vi "Coord window-PictureMap zoom to fit.vi"(8 "error in":errorcluster, 10 "Conditional?":bool) -> (0 "error out":errorcluster)   [LabVIEW 2013]
uses:
  Globals/Coord window-Globals.vi
panel:
  # "ZOOM TO FIT"
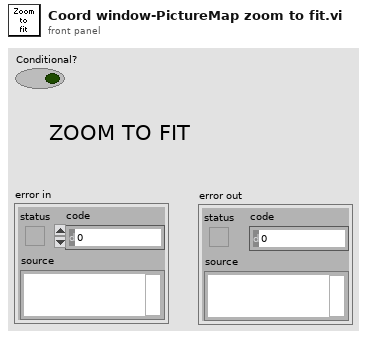
[diagram p1: front panel]
types:
  T1 = typedef "Coordinate list window refs.ctl" = cluster{"Window Name (i.e. Key)":string, "menu reference":refnum<k9>, "VI's reference":refnum<vi>, "Pane 1":refnum<vi>, "Pane 2":refnum<vi>, "Coord Listbox":refnum<vi>, "File name":refnum<vi>, "Picture Map":refnum<vi>, "Stage XYZ Position ind.":refnum<vi>}
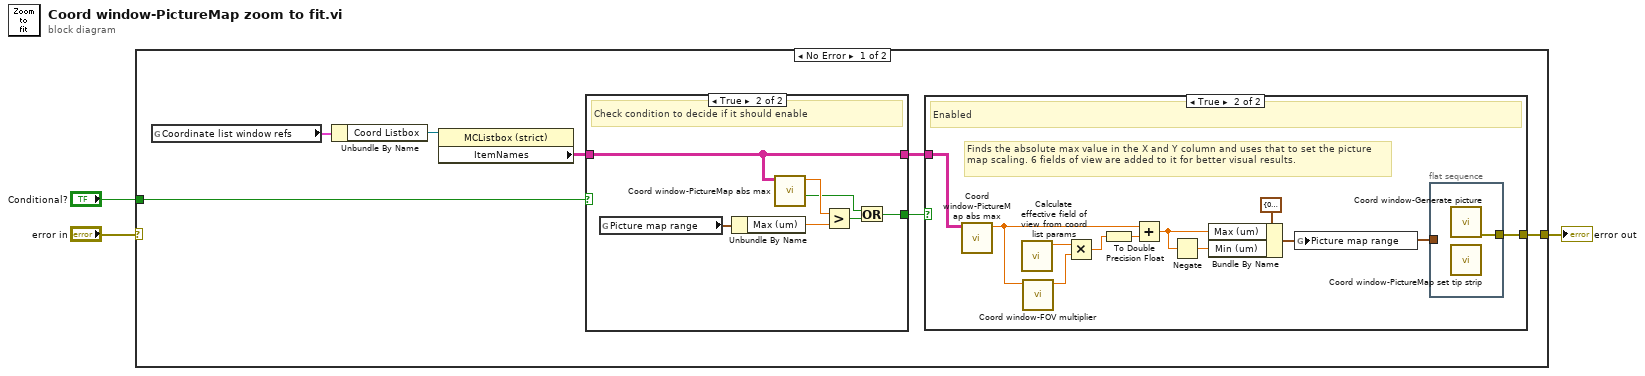
[diagram p0: block diagram]
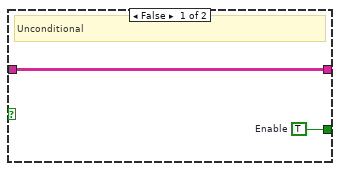
[diagram p2: hidden frame]
diagram:
  n1 = case shown="No Error" "error in" {
    selector: "error in" -> [_ w32]
    tunnel: [w5 w32] -> w2
    tunnel: "Conditional?" -> [w4 _]
    frame No Error {
      n2 = global read "Coord window-Globals.vi" "Coordinate list window refs"() -> (w8:T1)
      n3 = Unbundle By Name(w8) -> ("Coord Listbox"=w9:refnum<vi>)
      n4 = property on="Property Node" class="MCListbox (strict)"(reference=w9) -> ("ItemNames"=w7:string[][])  [unwired: 1 in, 2 out]
      n5 = case shown="True" w4 {
        tunnel: [w11 w14] -> w10
        tunnel: w7 -> [w12 w16]
        tunnel: [w12 w16] -> w6
        frame False {
          w11 = TRUE  # Enable
          # "Unconditional"
        }
        frame True {
          # "Check condition to decide if it should enable"
          n6 = global read "Coord window-Globals.vi" "Picture map range"() -> (w18:cluster{"Min (um)":dbl, "Max (um)":dbl})
          n7 = Unbundle By Name(w18) -> ("Max (um)"=w17:dbl)
          n8 = call "Coord window-PictureMap abs max.vi"("Coordinates Listbox Item Names"=w16) -> ("Auto-scale"=w13:bool, "Absolute maximum coordinate (inc current position)"=w19:dbl)  [unwired: 9 in]
          n9 = Greater?(x=w19, y=w17) -> (0:w15:bool)
          n10 = Or(x=w13, y=w15) -> (x .or. y?=w14:bool)
        }
      }
      n11 = case shown="True" w10 {
        tunnel: w6 -> [_ w24]
        tunnel: [_ w23] -> w5
        frame False {
          # "Disabled"
        }
        frame True {
          # "Finds the absolute max value in the X and Y column and uses that to set the picture map scaling. 6 fields of view are added to it for better visual results."
          # "Enabled"
          n12 = call "Coord window-PictureMap abs max.vi"("Coordinates Listbox Item Names"=w24) -> ("Absolute maximum coordinate (inc current position)"=w22:dbl)  [unwired: 9 in, 1 out]
          n13 = call "Calculate effective field of view from coord list params.vi"() -> ("Effective FOV (um)"=w20:sgl)  [unwired: 11 in]
          n14 = call "Coord window-FOV multiplier.vi"("Absolute maximum coordinate"=w22) -> ("Field of view multiplier"=w21:sgl)  [unwired: 10 in]
          n15 = Multiply(x=w20, y=w21) -> (x*y=w25:sgl)
          n16 = To Double Precision Float(number=w25) -> (double precision float=w27:dbl)
          n17 = Add(x=w22, y=w27) -> (x+y=w28:dbl)
          n18 = Negate(x=w28) -> (-x=w29:dbl)
          n19 = Bundle By Name(cluster=cluster{"Min (um)":dbl, "Max (um)":dbl} {"Min (um)"=0.0, "Max (um)"=0.0} ("Picture map range"), "Max (um)"=w28, "Min (um)"=w29) -> (w26:cluster{"Min (um)":dbl, "Max (um)":dbl})
          n20 = global write "Coord window-Globals.vi" "Picture map range"(w26) -> ()
          n21 = flat-sequence {
            tunnel: w26 -> [_]
            tunnel: [w31] -> w23
            frame #0 {
              n22 = call "Coord window-Generate picture.vi"() -> ("error out"=w31:errorcluster)  [unwired: 11 in]
              n23 = call "Coord window-PictureMap set tip strip.vi"() -> ()  [unwired: 12 in]
            }
          }
        }
      }
    }
    frame Error {
    }
  }
  "error out" <- w2
